vi "PWMSub.vi"(8 "FPGA I/O In":refnum<k21>="ConnectorC/DIO5", 10 "Pluse":u32, 11 "Count(Ticks)":u32 caption="Hz") -> ()   [LabVIEW 2018]
uses:
  <vilib>/rvi/eio/common/nirviEmuTemplateMethod_errors.vi
  <vilib>/eio/EIONode/EIONode.xnode
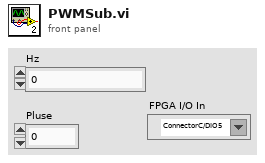
[diagram p1: front panel]
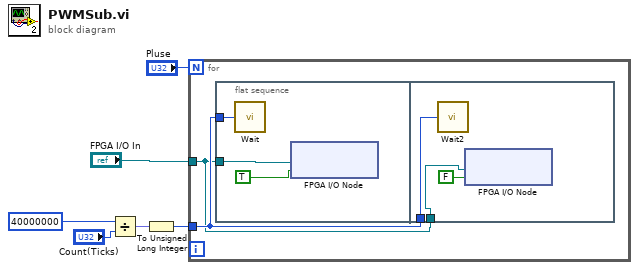
[diagram p0: block diagram]
diagram:
  n1 = Divide(x=u32 40000000, y="Count(Ticks)") -> (x/y=w6:fxp<+,32,16>)
  n2 = To Unsigned Long Integer(number=w6) -> (unsigned 32bit integer=w5:u32)
  n3 = for {
    N: "Pluse" -> [_]
    tunnel: w5 -> [w8]
    tunnel: "FPGA I/O In" -> [w7]
    n4 = flat-sequence {
      tunnel: w8 -> [w10]
      tunnel: w7 -> [w9]
      tunnel: w8 -> [w13]
      tunnel: w7 -> [w12]
      frame #0 {
        n5 = call "Wait"("Count(Ticks)"=w10) -> ()  [unwired: 1 out]
        n6 = xnode "FPGA I/O Node"("I/O Item"=TRUE ("ConnectorC/DIO5"), "FPGA I/O In"=w9) -> ()  [unwired: 1 out]
      }
      frame #1 {
        n7 = call "Wait2"("Count(Ticks)"=w13) -> ()  [unwired: 1 out]
        n8 = xnode "FPGA I/O Node"("I/O Item"=FALSE ("ConnectorC/DIO5"), "FPGA I/O In"=w12) -> ()  [unwired: 1 out]
      }
    }
  }
